vi "RFM Control and Status.LISR.Global Interrupt Enable.Get.vi"(8 "error in (no error)":errorcluster, 11 "GE 5565PIORC":refnum<class "GE 5565PIORC.lvclass">) -> (0 "error out":errorcluster, 2 "Global Interrupt Enable":bool, 3 "GE 5565PIORC out":refnum<class "GE 5565PIORC.lvclass">)   [LabVIEW 2016, in "GE 5565PIORC.lvclass"]
uses:
  GE 5565PIORC.lvclass
  Controls/Registers.RFM Control and Status.ctl
  GE 5565PIORC.lvclass/GE 5565PIORC.ctl
  <vilib>/Instr/_visa.llb/VISA Register Access Address Space.ctl
  Binary Operations/Get Bits U32.vi
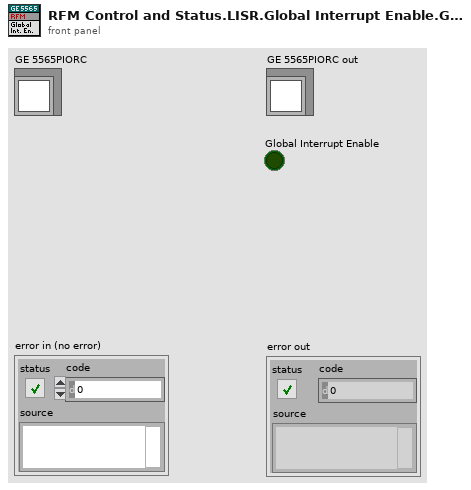
[diagram p1: front panel]
types:
  T1 = typedef "GE 5565PIORC.lvclass/Registers.RFM Control and Status.ctl" = enum16{"Board Revision", "Board ID", "Board Revision Build", "Node ID", "Local Control and Status", "Local Interrupt Status", "Local Interrupt Enable", "Network Target Data", "Network Target Node", "Network Interrupt Command", "Interrupt 1 Sender Data", "Interrupt 1 Sender ID", "Interrupt 2 Sender Data", "Interrupt 2 Sender ID", "Interrupt 3 Sender Data", "Interrupt 3 Sender ID", "Interrupt 4 Sender Data", "Interrupt 4 Sender ID"}
  T2 = typedef "VISA Register Access Address Space.ctl" = u16
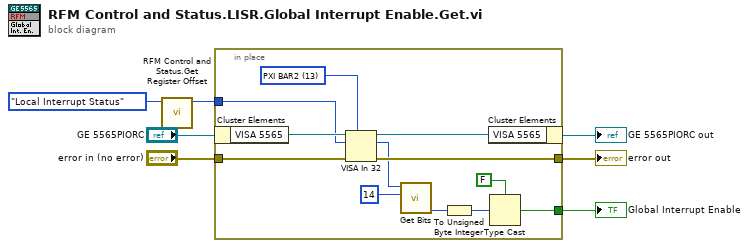
[diagram p0: block diagram]
diagram:
  n1 = call "RFM Control and Status.Get Register Offset.vi"("RFM Control and Status Register"=Registers.RFM_Control_and_Status."Local Interrupt Status") -> ("Offset"=w2:u32)  [unwired: 10 in]
  n2 = in-place {
    in-place-border: "error in (no error)" -> [w17]
    in-place-border: [w16] -> w5
    in-place-border: w2 -> [w12]
    in-place-border: [w8] -> w1
    w15 = T2 13 items=["VXI/VME A16"=1, "VXI/VME A24"=2, "VXI/VME A32"=3, "VXI/VME A64"=4, "PXI Memory Allocations"=9, "PXI Configuration"=10, "PXI BAR0"=11, "PXI BAR1"=12, "PXI BAR2"=13, "PXI BAR3"=14, "PXI BAR4"=15, "PXI BAR5"=16] ("Address Space")
    n3 = in-place-cluster #1("GE 5565PIORC") -> ("VISA 5565"=w19:refnum<visa-resource-name>)
    n4 = VISA In 32(7:w15, 8:w17, 10:w12, 11:w19) -> (0:w16:errorcluster, 2:w14:u32, 3:w18:refnum<visa-resource-name>)
    n5 = call-poly "Get Bits.vi"("Start Index (0)"=u8 14, "Register in"=w14) -> ("Value"=w9:u32)  [unwired: 6 in, 3 out]
    n6 = To Unsigned Byte Integer(number=w9) -> (unsigned 8bit integer=w11:u8)
    n7 = in-place-cluster #1("VISA 5565"=w18) -> (→"GE 5565PIORC out":refnum<class "GE 5565PIORC.lvclass">)
    n8 = Type Cast(type=FALSE, x=w11) -> (*(type *) &x=w8:bool)
  }
  "error out" <- w5
  "Global Interrupt Enable" <- w1
